vi "Process Async.vi"(9 "HTTPS?":bool, 10 "Connection":refnum<class "HTTP TCP Client.lvclass">, 11 "Server in":refnum<class "Server.lvclass">) -> ()   [LabVIEW 2020, in "HTTP Server.lvlib" / "Server.lvclass"]
uses:
  Server.lvclass
  HTTP TCP Client/HTTP TCP Client.lvclass
  C:/dev/lv20CE/relink/lv-stream/stream/Connection/Connection.lvclass
  C:/dev/lv20CE/relink/lv-stream/stream/Endpoint/Endpoint.lvclass
  Server.lvclass/Server.ctl
  Processing/Processing.lvclass/Processing.ctl
  lv-stream/stream/Endpoint/Endpoint.lvclass
  RequestTraceLog/RequestTraceLog.lvclass
  Processing/Processing.lvclass
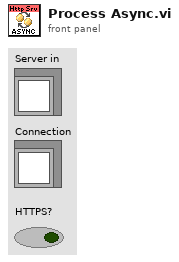
[diagram p1: front panel]
types:
  T1 = typedef "HTTP Server.lvlib/Server.lvclass/Ref Data.ctl" = cluster{"Connection Handler Map":T2, "Request Handler Map":T4, "Route Handler Map":T5, "Controller Handler Map":T6, "Controller Map":T7, "Response Handler Map":T8, "Complete Handler Map":T9, "Exception Handler Map":T10, "Connection Handler Index":u16, "Request Handler Index":u16, "Route Handler Index":u16, "Controller Handler Index":u16, "Controller Index":u16, "Response Handler Index":u16, "Complete Handler Index":u16, "Exception Handler Index":u16, "Values":refnum<class "Values.lvclass">, "Path":path, "Session Type":refnum<class "Session.lvclass">, "Session Cookie Name":string, "WebSocket Handler":refnum<class "WebSocket Handler.lvclass">, "WebSocket Handling":bool}
  T2 = typedef "HTTP Server.lvlib/Connection Handler Map.ctl" = map{T3, refnum<class "Connection Handler.lvclass">}
  T3 = typedef "HTTP Server.lvlib/Priority.ctl" = cluster{"Entity":u16, "Index":u16}
  T4 = typedef "HTTP Server.lvlib/Request Handler Map.ctl" = map{T3, refnum<class "Request Handler.lvclass">}
  T5 = typedef "HTTP Server.lvlib/Route Handler Map.ctl" = map{T3, refnum<class "Route Handler.lvclass">}
  T6 = typedef "HTTP Server.lvlib/Controller Handler Map.ctl" = map{T3, refnum<class "Controller Handler.lvclass">}
  T7 = typedef "HTTP Server.lvlib/Controller Map.ctl" = map{T3, refnum<class "Controller.lvclass">}
  T8 = typedef "HTTP Server.lvlib/Response Handler Map.ctl" = map{T3, refnum<class "Response Handler.lvclass">}
  T9 = typedef "HTTP Server.lvlib/Complete Handler Map.ctl" = map{T3, refnum<class "Complete Handler.lvclass">}
  T10 = typedef "HTTP Server.lvlib/Exception Handler Map.ctl" = map{T3, refnum<class "Exception Handler.lvclass">}
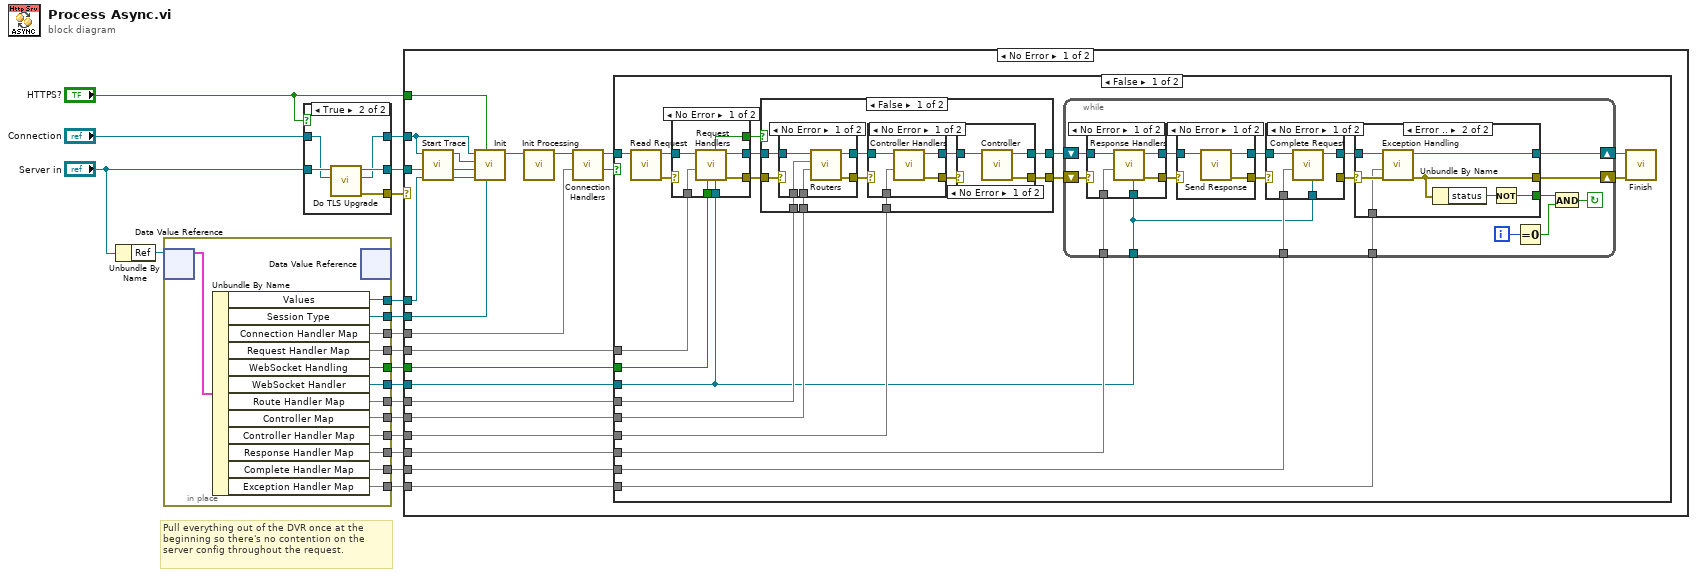
[diagram p0: block diagram]
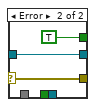
[diagram p6: hidden frame]
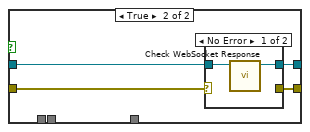
[diagram p10: hidden frame]
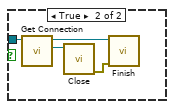
[diagram p12: hidden frame]
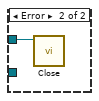
[diagram p13: hidden frame]
diagram:
  # "Pull everything out of the DVR once at the beginning so there's no contention on the server config throughout the request."
  n1 = Unbundle By Name("Server in") -> ("Ref"=w14:refnum<data-value>)
  n2 = in-place {
    in-place-border: [w31] -> w13
    in-place-border: [w30] -> w12
    in-place-border: [w23] -> w11
    in-place-border: [w29] -> w10
    in-place-border: [w28] -> w9
    in-place-border: [w27] -> w8
    in-place-border: [w26] -> w7
    in-place-border: [w25] -> w6
    in-place-border: [w24] -> w5
    in-place-border: [w22] -> w4
    in-place-border: [w21] -> w3
    in-place-border: [w20] -> w2
    n3 = in-place-dvr #1(w14) -> (w32:T1)  [unwired: 1 out]
    n4 = Unbundle By Name(w32) -> ("Values"=w20:refnum<class "Values.lvclass">, "Session Type"=w24:refnum<class "Session.lvclass">, "Connection Handler Map"=w31:T2, "Request Handler Map"=w30:T4, "WebSocket Handling"=w22:bool, "WebSocket Handler"=w21:refnum<class "WebSocket Handler.lvclass">, "Route Handler Map"=w23:T5, "Controller Map"=w29:T7, "Controller Handler Map"=w28:T6, "Response Handler Map"=w27:T8, "Complete Handler Map"=w26:T9, "Exception Handler Map"=w25:T10)
    n5 = in-place-dvr #1() -> ()  [unwired: 1 in, 2 out]
  }
  n6 = case shown="True" "HTTPS?" {
    tunnel: "Server in" -> [w34 w39]
    tunnel: [w34 w38] -> w19
    tunnel: "Connection" -> [w33 w37]
    tunnel: [w33 w36] -> w17
    tunnel: [_ w35] -> w15
    frame False {
    }
    frame True {
      n7 = call "Do TLS Upgrade.vi"("Connection In"=w37, "Server in"=w39) -> ("error out"=w35:errorcluster, "Connection"=w36:refnum<class "HTTP TCP Client.lvclass">, "Server out"=w38:refnum<class "Server.lvclass">)  [unwired: 7 in]
    }
  }
  n8 = case shown="No Error" w15 {
    tunnel: w19 -> [w54 _]
    tunnel: w17 -> [w53 w175]
    tunnel: "HTTPS?" -> [w52 _]
    tunnel: w13 -> [w51 _]
    tunnel: w12 -> [w50 _]
    tunnel: w11 -> [w49 _]
    tunnel: w10 -> [w48 _]
    tunnel: w9 -> [w47 _]
    tunnel: w8 -> [w46 _]
    tunnel: w7 -> [w45 _]
    tunnel: w6 -> [w44 _]
    tunnel: w5 -> [w43 _]
    tunnel: w4 -> [w42 _]
    tunnel: w3 -> [w41 _]
    tunnel: w2 -> [w40 _]
    frame No Error {
      n9 = call "Start Trace.vi"("Connection"=w53) -> ("RequestTraceLog out"=w56:refnum<class "RequestTraceLog.lvclass">)  [unwired: 9 in, 1 out]
      n10 = call "Init.vi"("Session"=w43, "HTTPS?"=w52, "Values"=w40, "Server"=w54, "Trace Log"=w56, "Connection"=w53) -> ("Processing out"=w55:refnum<class "Processing.lvclass">)  [unwired: 5 in]
      n11 = call "Init Processing.vi"("Processing In"=w55) -> ("Processing"=w57:refnum<class "Processing.lvclass">)  [unwired: 10 in]
      n12 = call "Connection Handlers.vi"("Connection Handler Map"=w51, "Processing In"=w57) -> ("Close?"=w58:bool, "HTTP Server.lvlib:Processing"=w59:refnum<class "Processing.lvclass">)  [unwired: 8 in]
      n13 = case shown="False" w58 {
        tunnel: w50 -> [w78 _]
        tunnel: w49 -> [w75 _]
        tunnel: w48 -> [w74 _]
        tunnel: w47 -> [w73 _]
        tunnel: w46 -> [w72 _]
        tunnel: w45 -> [w71 _]
        tunnel: w44 -> [w70 _]
        tunnel: w59 -> [w69 w174]
        tunnel: w42 -> [w63 _]
        tunnel: w41 -> [w62 _]
        frame False {
          n14 = call "Read Request.vi"("Processing In"=w69) -> ("error out"=w68:errorcluster, "HTTP Server.lvlib:Processing"=w60:refnum<class "Processing.lvclass">)  [unwired: 9 in]
          n15 = case shown="No Error" w68 {
            selector: w68 -> [_ w133]
            tunnel: w78 -> [w129 _]
            tunnel: [w128 w133] -> w76
            tunnel: [w126 TRUE ("Early Response?")] -> w77
            tunnel: w60 -> [w130 w132]
            tunnel: [w127 w132] -> w67
            tunnel: w63 -> [w125 _]
            tunnel: w62 -> [w124 _]
            frame No Error {
              n16 = call "Request Handlers.vi"("WebSocket Handler"=w124, "WebSocket Handling"=w125, "Request Handler Map"=w129, "Processing In"=w130) -> ("error out"=w128:errorcluster, "HTTP Server.lvlib:Processing"=w127:refnum<class "Processing.lvclass">, "Early Response?"=w126:bool)  [unwired: 5 in]
            }
            frame Error {
            }
          }
          n17 = case shown="False" w77 {
            tunnel: w76 -> [w144 w165]
            tunnel: w75 -> [w140 _]
            tunnel: w74 -> [w139 _]
            tunnel: w73 -> [w142 _]
            tunnel: w67 -> [w141 w166]
            tunnel: [w135 w164] -> w66
            tunnel: [w134 w163] -> w65
            frame False {
              n18 = case shown="No Error" w144 {
                selector: w144 -> [_ w151]
                tunnel: [w146 w151] -> w143
                tunnel: w141 -> [w149 w150]
                tunnel: w140 -> [w148 _]
                tunnel: w139 -> [w147 _]
                tunnel: [w145 w150] -> w138
                frame No Error {
                  n19 = call "Routers.vi"("Controller Map"=w147, "Route Handler Map"=w148, "Processing In"=w149) -> ("error out"=w146:errorcluster, "Processing"=w145:refnum<class "Processing.lvclass">)  [unwired: 7 in]
                }
                frame Error {
                }
              }
              n20 = case shown="No Error" w143 {
                selector: w143 -> [_ w157]
                tunnel: w142 -> [w154 _]
                tunnel: w138 -> [w155 w156]
                tunnel: [w153 w157] -> w137
                tunnel: [w152 w156] -> w136
                frame No Error {
                  n21 = call "Controller Handlers.vi"("Controller Handler Map"=w154, "Processing In"=w155) -> ("error out"=w153:errorcluster, "Processing"=w152:refnum<class "Processing.lvclass">)  [unwired: 8 in]
                }
                frame Error {
                }
              }
              n22 = case shown="No Error" w137 {
                selector: w137 -> [_ w162]
                tunnel: w136 -> [w160 w161]
                tunnel: [w159 w162] -> w135
                tunnel: [w158 w161] -> w134
                frame No Error {
                  n23 = call "Controller.vi"("Processing In"=w160) -> ("error out"=w159:errorcluster, "Processing"=w158:refnum<class "Processing.lvclass">)  [unwired: 9 in]
                }
                frame Error {
                }
              }
            }
            frame True {
              n24 = case shown="No Error" w165 {
                selector: w165 -> [_ w170]
                tunnel: w166 -> [w168 w169]
                tunnel: [_ w170] -> w164
                tunnel: [w167 w169] -> w163
                frame No Error {
                  n25 = call "Check WebSocket Response.vi"("Processing In"=w168) -> ("Processing"=w167:refnum<class "Processing.lvclass">)  [unwired: 10 in]
                }
                frame Error {
                }
              }
            }
          }
          n26 = while {
            tunnel: w72 -> [w96]
            tunnel: w71 -> [w94]
            tunnel: w70 -> [w93]
            tunnel: w62 -> [w83]
            shift-right: [w84] -> w64
            shift-left: w66 -> [w91]
            shift-right: [w85] -> w61
            shift-left: w65 -> [w90]
            i -> [w80]
            stop <- w81 continue-if-true
            n27 = case shown="No Error" w91 {
              selector: w91 -> [_ w103]
              tunnel: w96 -> [w100 _]
              tunnel: [w99 w103] -> w95
              tunnel: w90 -> [w101 w102]
              tunnel: [w98 w102] -> w89
              tunnel: w83 -> [w97 _]
              frame No Error {
                n28 = call "Response Handlers.vi"("WebSocket Handler"=w97, "Response Handler Map"=w100, "Processing In"=w101) -> ("error out"=w99:errorcluster, "HTTP Server.lvlib:Processing"=w98:refnum<class "Processing.lvclass">)  [unwired: 7 in]
              }
              frame Error {
              }
            }
            n29 = case shown="No Error" w95 {
              selector: w95 -> [_ w108]
              tunnel: [w105 w108] -> w92
              tunnel: w89 -> [w106 w107]
              tunnel: [w104 w107] -> w88
              frame No Error {
                n30 = call "Send Response.vi"("Processing In"=w106) -> ("error out"=w105:errorcluster, "HTTP Server.lvlib:Processing"=w104:refnum<class "Processing.lvclass">)  [unwired: 9 in]
              }
              frame Error {
              }
            }
            n31 = case shown="No Error" w92 {
              selector: w92 -> [_ w114]
              tunnel: w94 -> [w112 _]
              tunnel: [_ w114] -> w87
              tunnel: w88 -> [w111 w113]
              tunnel: [w110 w113] -> w86
              tunnel: w83 -> [w109 _]
              frame No Error {
                n32 = call "Complete Request.vi"("WebSocket Handler"=w109, "Complete Handler Map"=w112, "Processing In"=w111) -> ("HTTP Server.lvlib:Processing"=w110:refnum<class "Processing.lvclass">)  [unwired: 8 in]
              }
              frame Error {
              }
            }
            n33 = case shown="Error .." w87 {
              selector: w87 -> [w116 w122]
              tunnel: w93 -> [_ w121]
              tunnel: w86 -> [w115 w123]
              tunnel: [w115 w120] -> w85
              tunnel: [w116 w119] -> w84
              tunnel: [_ w117] -> w82
              frame No Error {
              }
              frame Error {
                n34 = call "Exception Handling.vi"("error in (no error)"=w122, "Exception Handler Map"=w121, "Processing In"=w123) -> ("error out"=w119:errorcluster, "HTTP Server.lvlib:Processing"=w120:refnum<class "Processing.lvclass">)  [unwired: 7 in]
                n35 = Unbundle By Name(w119) -> ("status"=w118:bool)
                n36 = Not(x=w118) -> (.not. x?=w117:bool)
              }
            }
            n37 = Equal To 0?(x=w80) -> (x = 0?=w79:bool)
            n38 = And(x=w82, y=w79) -> (x .and. y?=w81:bool)
          }
          n39 = call "Finish.vi"("error in (no error)"=w64, "Processing"=w61) -> ()  [unwired: 10 in]
        }
        frame True {
          n40 = call "Get Connection.vi"("Processing in"=w174) -> ("Connection"=w173:refnum<class "HTTP TCP Client.lvclass">, "Processing out"=w172:refnum<class "Processing.lvclass">)  [unwired: 9 in]
          n41 = call "Close.vi"("Endpoint in"=w173) -> ("error out"=w171:errorcluster)  [unwired: 9 in, 1 out]
          n42 = call "Finish.vi"("error in (no error)"=w171, "Processing"=w172) -> ()  [unwired: 10 in]
        }
      }
    }
    frame Error {
      n43 = call "Close.vi"("Endpoint in"=w175) -> ()  [unwired: 9 in, 2 out]
    }
  }
